vi "Konfig AK.vi"() -> ()   [LabVIEW 2020, in "AK-Schnittstelle.lvlib"]
uses:
  AK-Schnittstelle.lvlib
  Visualisierungs Elemente/VISA Control.ctl
  Seriell - Parity Bits.ctl
  Seriell - Stop Bits.ctl
  Seriell - Flow Control.ctl
  Visualisierungs Elemente/Button.ctl
  Seriell - Baud Rate.ctl
  Seriell - Data Bits.ctl
  Visualisierungs Elemente/String - Ausgabefeld.ctl
  AK Befehlssatz.ctl
  Aktionen Gespeicherte Werte.ctl
  Seiten/FT-IR/FGV FT-IR Gasliste Aktionen.ctl
  AK Namen Aktionen.ctl
  Daten weitergeben Aktionen.ctl
  SysLog/SysLog Interface.ctl
  Seiten/FT-IR/FT-IR.lvlib
  Allgemein/allgemeine Sub-VIs.lvlib
  Sprachverwaltung/Sprachverwaltung.lvlib
  SysLog/SysLog.lvlib
  <vilib>/Utility/Data Type/NI_Data Type.lvlib
  AK Seriell/AK Seriell.lvlib
panel:
  in  "Registerkarte":T1(tab)
  in  "Nur im Messen übertragen":bool caption="Loggen?"
  in  "AK Befehlssatz":T2=enum."AVL (Puma)"
  in  "Timeout":u16
  in  "Loggen?":bool
  in  "data bits":T3=8 items=["8"=8, "7"=7, "6"=6, "5"=5, "4"=4]
  in  "Baud Rate":T4=38400 items=["38400"=38400, "19200"=19200, "14400"=14400, "9600"=9600, "4800"=4800, "2400"=2400]
  in  "TCP aktiv":bool
  in  "Seriell aktiv":bool
  in  "Port":u16
  in  "flow control":T5 items=["None"=0, "XON/XOFF"=1, "RTS/CTS"=2, "DTR/DSR"=4]
  in  "stop bits":T6=10 items=["1.0"=10, "1.5"=15, "2.0"=20]
  in  "parity":T7 items=["None", "Odd", "Even", "Mark", "Space"]
  in  "VISA resource name":T8="COM1"
  out "EKFG vom Host":string[](array[string])
  in  "Original Liste":i32(listbox)
  in  "Konfigurierte Liste":i32(listbox)
  in  "Übernehmen":T9
  in  "Löschen":T9
  in  "Alle Löschen":T9
  in  "AK Namen":T10[](array[typedef])
  out "Gasliste":T10[](array[typedef])
  in  "Neuer Eintrag":T9
  out "Empfangspuffer":string[](array[string])
  out "Antwort":string[](array[string])
  out "Details ALLE":string[](array[string])
  in  "ABBRECHEN":T9
  in  "Speichern":T9
  # "Konfiguration AK-Schnittstelle"
  # "Seriell"
  # "TCP"
  # "Serielle Schnittstelle:"
  # "Port:"
  # "Baud rate:"
  # "Timeout:"
  # "sec"
  # "Data bits:"
  # "Parity bits:"
  # "Stop bits:"
  # "Flow control:"
  # "Messwerte nur in Messen übertragen:"
  # "AK in Datei Loggen:"
  # "AK Befehlssatz:"
  # "Konfiguration Kanalreihenfolge (EKFG)"
  # "Konfiguration AK-Namen (für EKFG)"
  # "Gasliste"
  # "AK Namen"
  # "Status AK-Kommunikation"
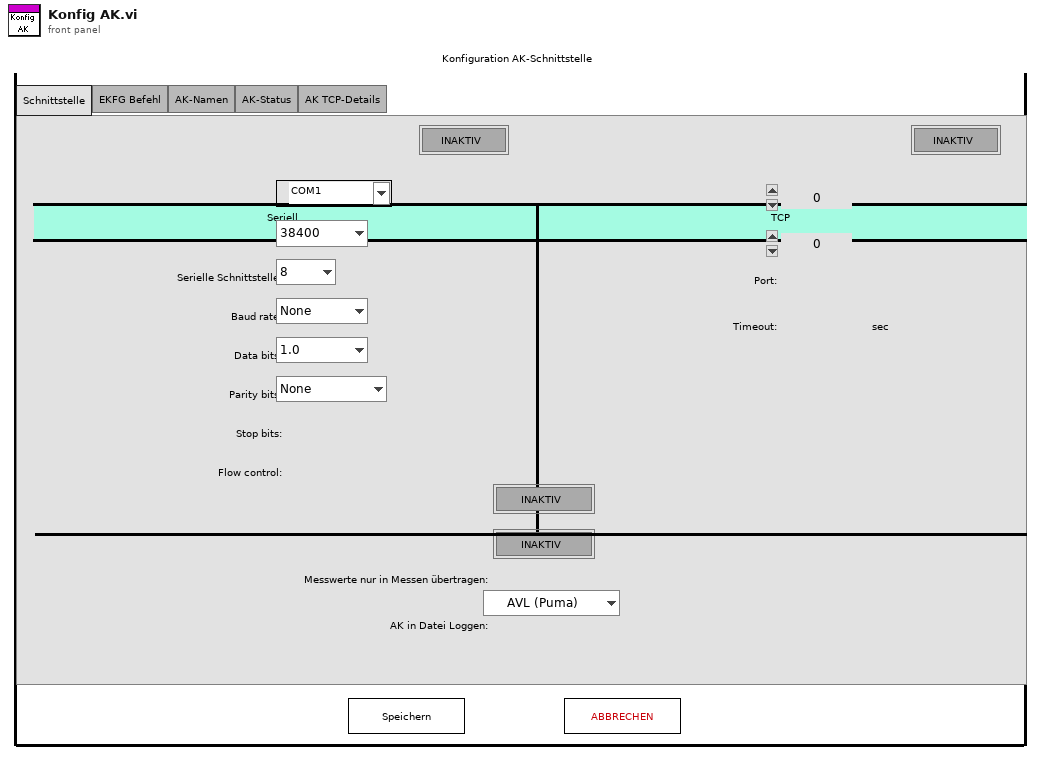
[diagram p1: front panel]
types:
  T1 = enum32{"Interface", "EKFG Commando", "AK-Name", "AK-Status", "AK TCP-Details"}
  T2 = typedef "AK-Schnittstelle.lvlib/AK Befehlssatz.ctl" = enum16{"MEXA", "IAG v1.4", "AVL (Puma)", "PEUS"}
  T3 = typedef "AK-Schnittstelle.lvlib/AK Seriell.lvlib/Seriell - Data Bits.ctl" = u16
  T4 = typedef "AK-Schnittstelle.lvlib/AK Seriell.lvlib/Seriell - Baud Rate.ctl" = u16
  T5 = typedef "AK-Schnittstelle.lvlib/AK Seriell.lvlib/Seriell - Flow Control.ctl" = u16
  T6 = typedef "AK-Schnittstelle.lvlib/AK Seriell.lvlib/Seriell - Stop Bits.ctl" = u16
  T7 = typedef "AK-Schnittstelle.lvlib/AK Seriell.lvlib/Seriell - Parity Bits.ctl" = u16
  T8 = typedef "VISA Control.ctl" = refnum<visa-resource-name>
  T9 = typedef "Button.ctl" = bool
  T10 = typedef "String - Ausgabefeld.ctl" = string
  T11 = typedef "FT-IR.lvlib/FGV FT-IR Gasliste Aktionen.ctl" = enum16{"lesen", "Gasliste FT-IR", "Gasliste ausgelesen", "laden", "speichern", "löschen"}
  T12 = typedef "AK-Schnittstelle.lvlib/AK Namen Aktionen.ctl" = enum16{"lesen", "laden", "speichern Namen", "AK Namen", "Liste erstellen", "EKFG erstellen", "speichern EKFG", "EKFG schreiben", "Neuen Eintrag erzeugen"}
  T13 = typedef "AK-Schnittstelle.lvlib/Aktionen Gespeicherte Werte.ctl" = enum16{"lesen", "laden", "speichern", "Seriell", "TCP", "Diverse", "AKTIV", "AK-Namen"}
  T14 = typedef "AK-Schnittstelle.lvlib/Diverse gespeicherte Werte.ctl" = cluster{"Kalibriergaseingang":i16, "SamplePoint":i16, "CalGas zu PNS":i16, "Gas-Reihenfolge":i16[], "Zeit 0-Gas":sgl, "Zeit CalGas":sgl, "AK Befehlssatz":T2}
  T15 = typedef "AK-Schnittstelle.lvlib/AK TCP.lvlib/TCP Parameter.ctl" = cluster{"Port":u16, "Timeout":u16}
  T16 = typedef "AK-Schnittstelle.lvlib/AK Seriell.lvlib/Serielle Parameter.ctl" = cluster{"VISA resource name":refnum<visa-resource-name>, "baud rate":u32, "data bits":u16, "parity":u16, "stop bits":u16, "flow control":u16}
  T17 = typedef "AK-Schnittstelle.lvlib/Daten weitergeben Aktionen.ctl" = enum16{"lesen", "schreiben", "Log löschen", "Detail", "Detail löschen", "Speicher Freigeben"}
  T18 = typedef "SysLog.lvlib/SysLog Interface.ctl" = cluster{"FehlermeldungsCode":i32, "ErfolgsmeldungsCode":i32, "ParameterListenString":string, "Anzeige":bool, "SysLogIcon":enum16{"OK", "Warnung", "Fehler"}, "intern":bool}
  T19 = typedef "AK-Schnittstelle.lvlib/AK Namen Listen.ctl" = cluster{"Namen":string[], "AK Namen":string[]}
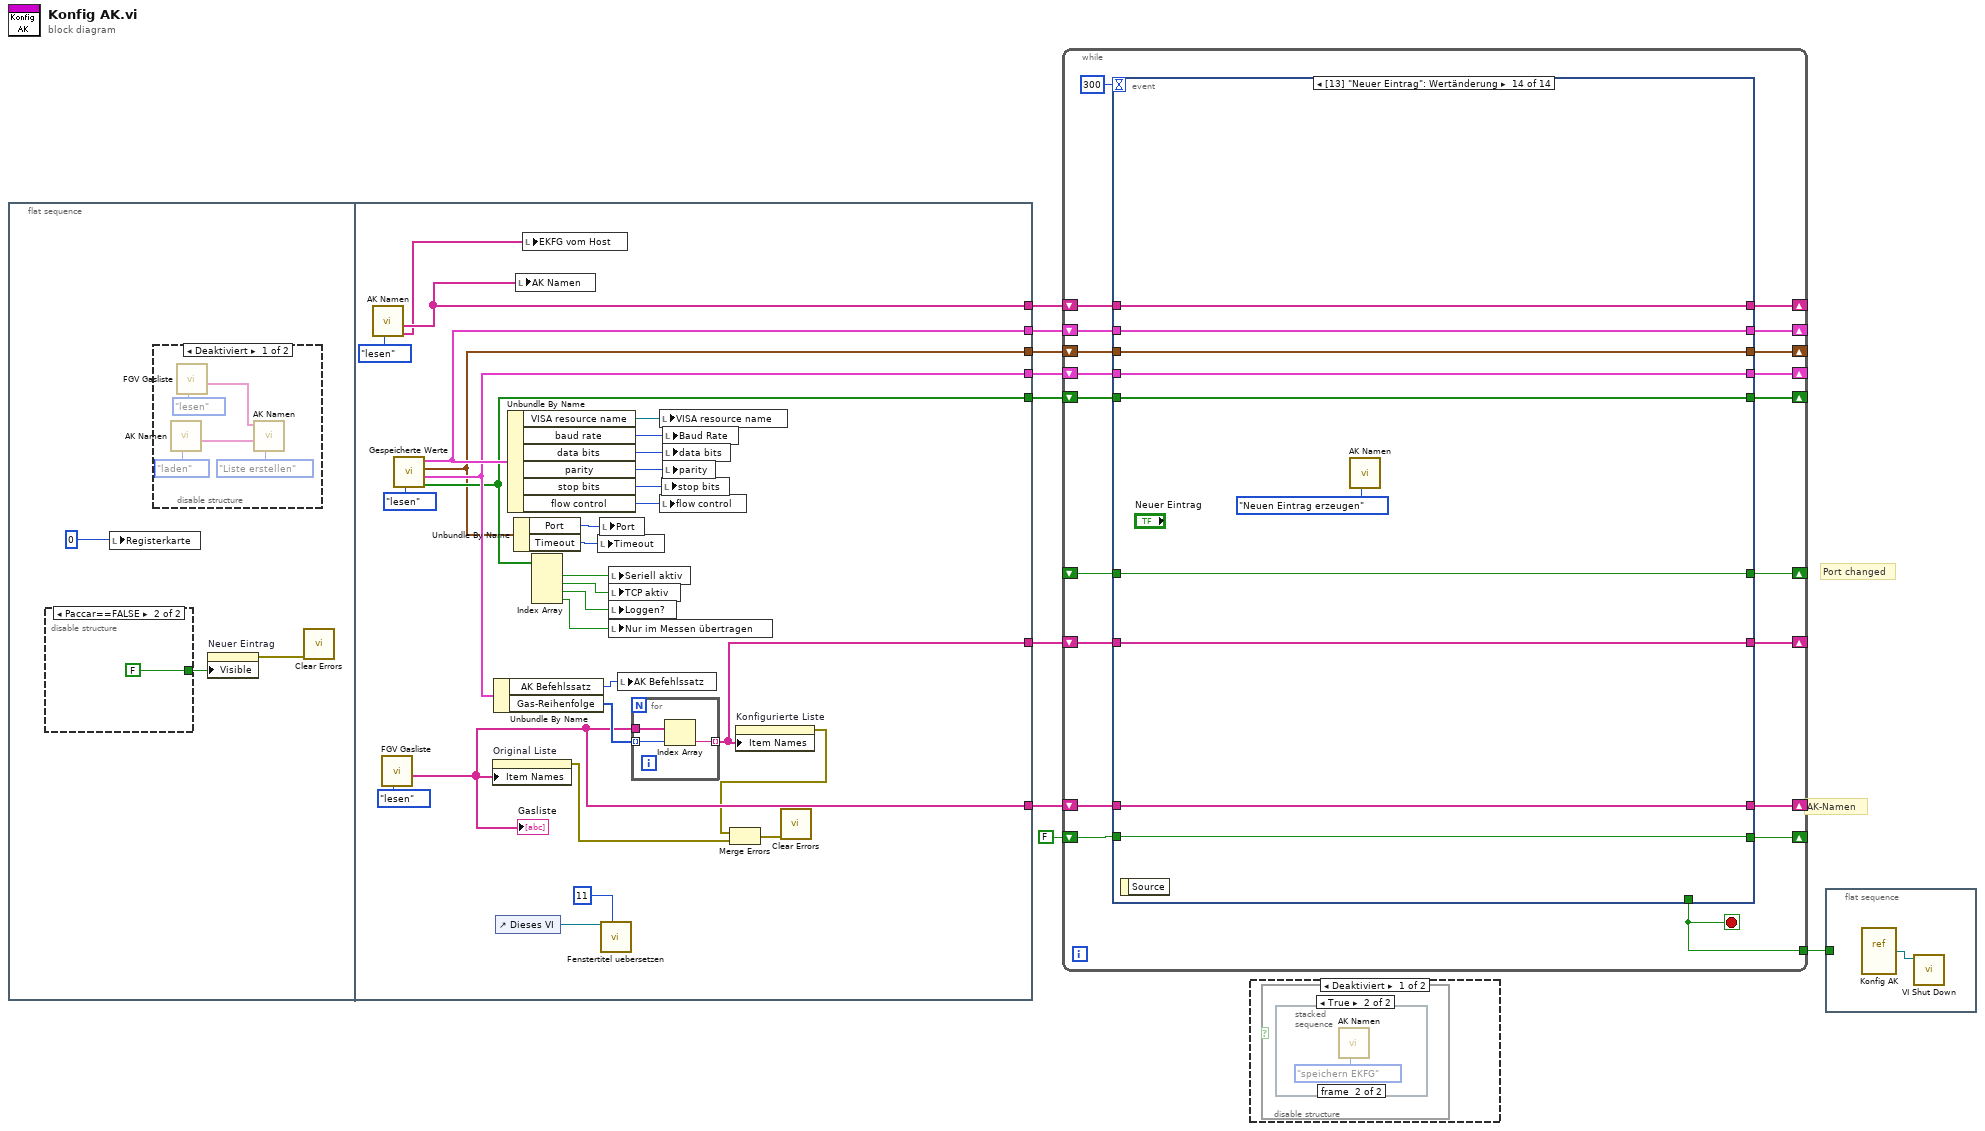
[diagram p0: block diagram]
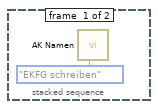
[diagram p3: hidden frame]
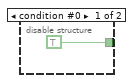
[diagram p5: hidden frame]
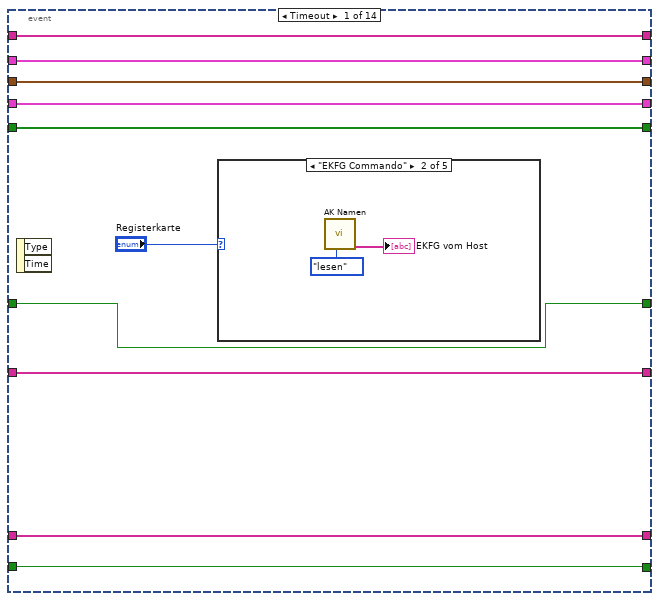
[diagram p7: hidden frame]
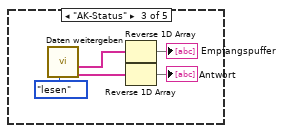
[diagram p9: hidden frame]
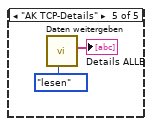
[diagram p11: hidden frame]
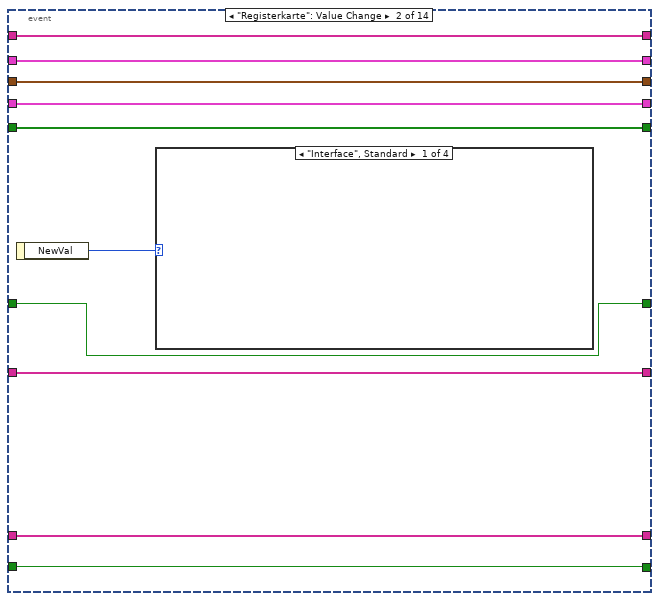
[diagram p12: hidden frame]
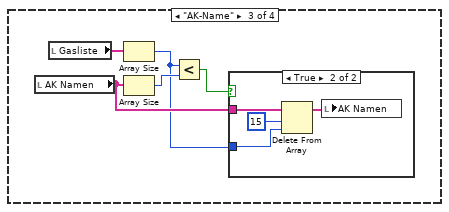
[diagram p14: hidden frame]
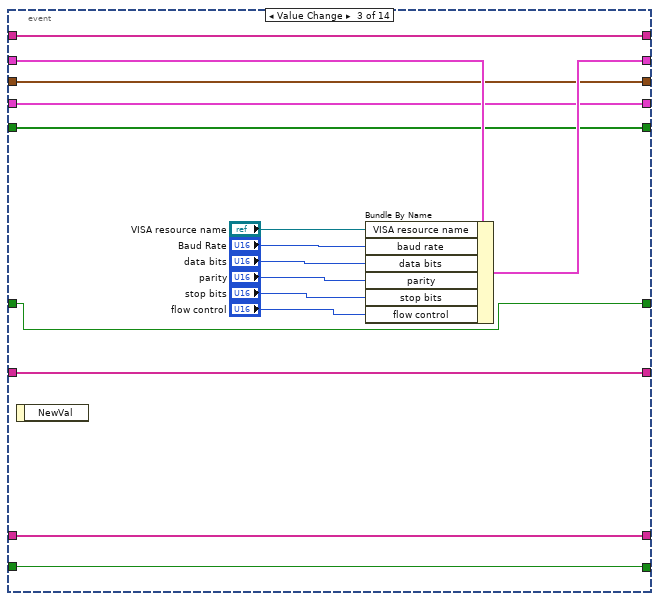
[diagram p17: hidden frame]
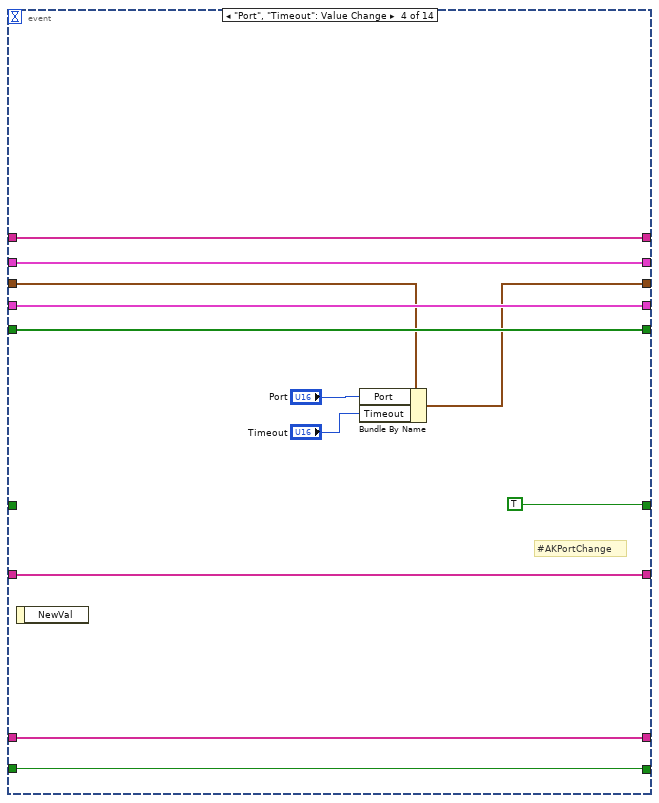
[diagram p18: hidden frame]
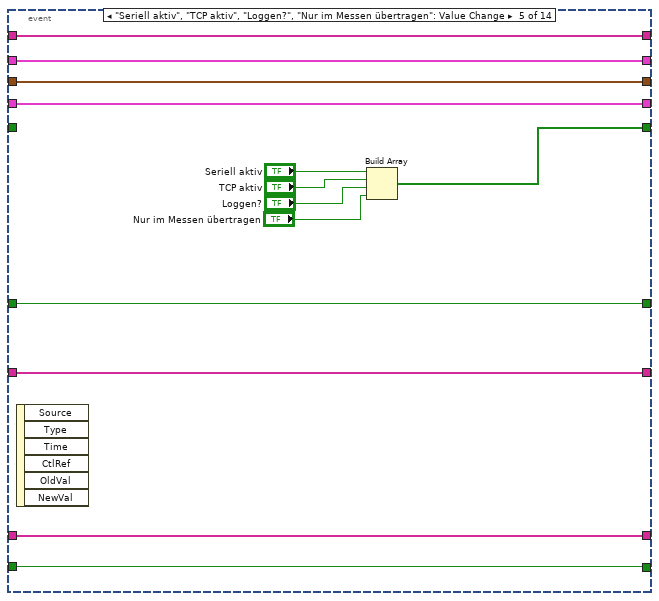
[diagram p19: hidden frame]
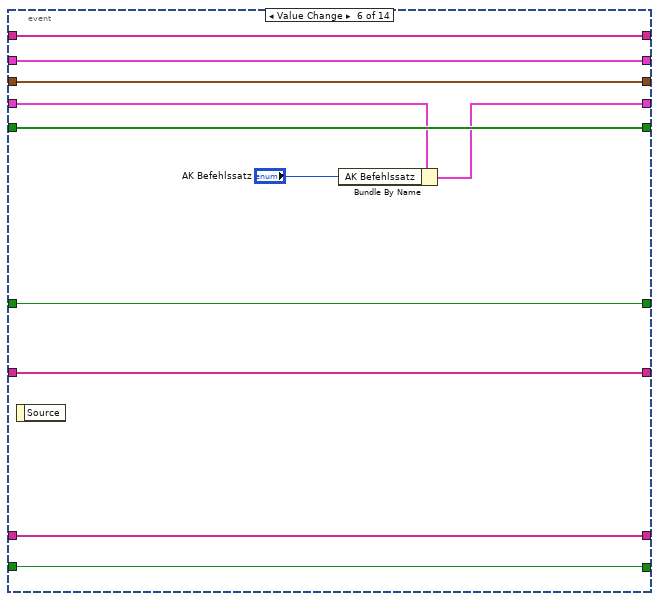
[diagram p20: hidden frame]
diagram:
  # "Port changed"
  # "AK-Namen"
  n1 = flat-sequence {
    tunnel: [w42] -> w9
    tunnel: [w33] -> w8
    tunnel: [w40] -> w7
    tunnel: [w38] -> w6
    tunnel: [w30] -> w4
    tunnel: [w35] -> w5
    tunnel: [w21] -> w3
    frame #0 {
      n2 = disable-structure shown="Paccar==FALSE" {
        disable-tunnel: [TRUE ("Sichtbar") FALSE ("Sichtbar")] -> w12
        frame condition #0 {
        }
        frame condition #1 (active) {
        }
      }
      n3 = local write "Registerkarte"(0) -> ()
      n4 = disable-structure shown="Deaktiviert" {
        frame Disabled {
          n5 = call "AK Namen.vi"("Aktionen"=AK_Namen_Aktionen."laden") -> ("AK Namen"=w17:string[])  [unwired: 7 in, 3 out]
          n6 = call "FGV Gasliste.vi"("Aktionen"=FGV_FT-IR_Gasliste_Aktionen."lesen") -> ("Aktuelle Gasliste gesamt"=w15:T10[])  [unwired: 8 in, 2 out]
          n7 = call "AK Namen.vi"("Aktionen"=AK_Namen_Aktionen."Liste erstellen", "AK Namen"=w17, "Aktuelle Gasliste FT-IR"=w15) -> ()  [unwired: 5 in, 4 out]
        }
        frame Enabled {
        }
      }
      n8 = property on="Neuer Eintrag" class="Bool."("Visible"=w12) -> (error out=w11:errorcluster)  [unwired: 2 in, 1 out]
      n9 = call <vilib>:"Clear Errors.vi"("error in (no error)"=w11) -> ()  [unwired: 5 in, 2 out]
    }
    frame #1 {
      n10 = call "AK Namen.vi"("Aktionen"=AK_Namen_Aktionen."lesen") -> ("EKFG Liste"=w20:string[], "AK Namen"=w21:string[])  [unwired: 7 in, 2 out]
      n11 = call "FGV Gasliste.vi"("Aktionen"=FGV_FT-IR_Gasliste_Aktionen."lesen") -> ("Aktuelle Gasliste gesamt"=w30:T10[])  [unwired: 8 in, 2 out]
      "Gasliste" <- w30
      n12 = call "Gespeicherte Werte.vi"("Aktionen"=Aktionen_Gespeicherte_Werte."lesen") -> ("AKTIV?"=w35:bool[], "Diverse Werte"=w40:T14, "TCP Parameter"=w33:T15, "Serielle Parameter"=w42:T16)  [unwired: 6 in, 1 out]
      n13 = property on="Original Liste" class="Listenfeld (strikt)"("Item Names"=w30) -> (error out=w27:errorcluster)  [unwired: 2 in, 1 out]
      n14 = Unbundle By Name(w40) -> ("AK Befehlssatz"=w29:T2, "Gas-Reihenfolge"=w39:i16[])
      n15 = control-ref of="Dieses VI"() -> (w24:refnum<vi>)
      n16 = Unbundle By Name(w42) -> ("VISA resource name"=w48:refnum<visa-resource-name>, "baud rate"=w47:u32, "data bits"=w46:u16, "parity"=w45:u16, "stop bits"=w44:u16, "flow control"=w43:u16)
      n17 = Unbundle By Name(w33) -> ("Port"=w32:u16, "Timeout"=w31:u16)
      n18 = local write "AK Namen"(w21) -> ()
      n19 = local write "EKFG vom Host"(w20) -> ()
      n20 = Index Array(array=w35) -> (element #1=w37:bool, element #2=w36:bool, element #3=w34:bool, element #4=w25:bool)  [unwired: 4 in]
      n21 = local write "Timeout"(w31) -> ()
      n22 = local write "Port"(w32) -> ()
      n23 = call "Fenstertitel uebersetzen.vi"("Index (Seite)"=11, "Dieses VI"=w24) -> ()  [unwired: 6 in, 4 out]
      n24 = local write "Seriell aktiv"(w37) -> ()
      n25 = local write "TCP aktiv"(w36) -> ()
      n26 = local write "Loggen?"(w34) -> ()
      n27 = local write "Nur im Messen übertragen"(w25) -> ()
      n28 = local write "AK Befehlssatz"(w29) -> ()
      n29 = for {
        tunnel: w39 -> [w52] mode=indexing
        tunnel: w30 -> [w51]
        tunnel: [w50] -> w38 mode=indexing
        n30 = Index Array(array=w51, index=w52) -> (element=w50:T10)
      }
      n31 = local write "VISA resource name"(w48) -> ()
      n32 = local write "flow control"(w43) -> ()
      n33 = local write "stop bits"(w44) -> ()
      n34 = local write "Baud Rate"(w47) -> ()
      n35 = local write "data bits"(w46) -> ()
      n36 = local write "parity"(w45) -> ()
      n37 = property on="Konfigurierte Liste" class="Listenfeld (strikt)"("Item Names"=w38) -> (error out=w28:errorcluster)  [unwired: 2 in, 1 out]
      n38 = Merge Errors(w28, w27) -> (w26:errorcluster)
      n39 = call <vilib>:"Clear Errors.vi"("error in (no error)"=w26) -> ()  [unwired: 5 in, 2 out]
    }
  }
  n40 = while {
    shift-right: [w70] -> _
    shift-left: w9 -> [w71]
    shift-right: [w67] -> _
    shift-left: w8 -> [w69]
    shift-right: [w66] -> _
    shift-left: w7 -> [w68]
    shift-right: [w64] -> _
    shift-left: w6 -> [w65]
    shift-right: [w62] -> _
    shift-left: w5 -> [w63]
    shift-right: [w61] -> _
    shift-left: w4 -> [w60]
    shift-right: [w58] -> _
    shift-left: w3 -> [w59]
    tunnel: [w57] -> w2
    shift-right: [w56] -> _
    shift-left: FALSE -> [w55]
    shift-right: [w54] -> _
    shift-left: _ -> [w53]
    stop <- w57 stop-if-true
    n41 = event shown="[13] \"Neuer Eintrag\": Wertänderung" {
      selector: _ -> [_ _ _ _ _ _ _ _ _ _ _ _ _ _]
      dyn-events: _ -> [_ _ _ _ _ _ _ _ _ _ _ _ _ _]
      timeout: 300 -> [_ _ _ _ _ _ _ _ _ _ _ _ _ _]
      tunnel: w71 -> [w82 w97 w126 w138 w148 w161 w176 w207 w221 w236 w253 w283 w309 w312]
      tunnel: [w82 w97 w125 w138 w148 w161 w176 w207 w221 w236 w253 w283 w309 w312] -> w70
      tunnel: [_ _ _ _ _ _ _ _ _ _ _ TRUE ("ABBRECHEN") TRUE ("ABBRECHEN") _] -> w57
      tunnel: w69 -> [w81 w96 w119 w133 w147 w160 w175 w206 w220 w235 w252 w282 w307 w313]
      tunnel: w68 -> [w80 w95 w120 w137 w146 w156 w172 w203 w217 w233 w251 w259 w306 w314]
      tunnel: [w81 w96 w119 w130 w147 w160 w175 w206 w220 w235 w252 w282 w307 w313] -> w67
      tunnel: [w80 w95 w120 w137 w146 w154 w171 w202 w216 w232 w251 w259 w306 w314] -> w66
      tunnel: w65 -> [w74 w100 w118 w136 w149 w158 w170 _ w219 _ w249 w277 w305 w316]
      tunnel: [w74 w100 w118 w136 w149 w158 w173 w205 w215 w231 w249 w277 w305 w316] -> w64
      tunnel: w63 -> [w79 w94 w117 w135 _ w159 w167 w201 w213 w230 w250 w274 w304 w315]
      tunnel: [w79 w94 w117 w135 w145 w159 w167 w201 w213 w230 w250 w274 w304 w315] -> w62
      tunnel: [w77 w99 w114 w134 w144 w157 w166 w200 w212 w229 w248 w273 w303 w317] -> w61
      tunnel: w60 -> [w77 w99 w114 w134 w144 w157 w166 w200 w212 w229 w248 w273 w303 w317]
      tunnel: w59 -> [w76 w98 w113 w129 w142 w162 w165 w199 w211 w228 _ w271 w302 w311]
      tunnel: [w76 w98 w113 w129 w142 w162 w165 w199 w211 w228 w242 w271 w302 w311] -> w58
      tunnel: [w75 w93 w112 w128 w140 w153 TRUE TRUE TRUE TRUE w241 w266 w301 w319] -> w56
      tunnel: w55 -> [w75 w93 w112 w128 w140 w153 _ _ _ _ w241 w266 w301 w319]
      tunnel: [w73 w92 w111 TRUE w139 w152 w163 w196 w208 w225 w240 FALSE w300 w318] -> w54
      tunnel: w53 -> [w73 w92 w111 _ w139 w152 w163 w196 w208 w225 w240 w260 w300 w318]
      event Timeout {
        n42 = event-data() -> ()  [unwired: 1 in, 2 out]
        n43 = case shown="\"EKFG Commando\"" "Registerkarte" {
          frame "Interface", Default {
          }
          frame "EKFG Commando" {
            n44 = call "AK Namen.vi"("Aktionen"=AK_Namen_Aktionen."lesen") -> ("EKFG Liste"=→"EKFG vom Host":string[])  [unwired: 7 in, 3 out]
          }
          frame "AK-Status" {
            n45 = call "Daten weitergeben.vi"("Aktionen"=Daten_weitergeben_Aktionen."lesen") -> ("Antwort"=w86:string[], "Empfangspuffer"=w88:string[])  [unwired: 6 in, 3 out]
            n46 = Reverse 1D Array(array=w88) -> (reversed array=→"Empfangspuffer":string[])
            n47 = Reverse 1D Array(array=w86) -> (reversed array=→"Antwort":string[])
          }
          frame "AK-Name" {
          }
          frame "AK TCP-Details" {
            n48 = call "Daten weitergeben.vi"("Aktionen"=Daten_weitergeben_Aktionen."lesen") -> ("Details ALLE"=→"Details ALLE":string[])  [unwired: 6 in, 4 out]
          }
        }
      }
      event "Registerkarte": Value Change {
        n49 = event-data() -> ("NewVal"=w101:T1)  [unwired: 1 in]
        n50 = case shown="\"Interface\", Standard" w101 {
          frame "Interface", Default {
          }
          frame "EKFG Commando" {
          }
          frame "AK-Name" {
            n51 = local read "AK Namen"() -> (w104:T10[])
            n52 = local read "Gasliste"() -> (w106:T10[])
            n53 = Array Size(array=w106) -> (size(s)=w103:i32)
            n54 = Array Size(array=w104) -> (size(s)=w105:i32)
            n55 = Less?(x=w103, y=w105) -> (x < y?=w102:bool)
            n56 = case shown="True" w102 {
              tunnel: w104 -> [_ w110]
              tunnel: w103 -> [_ w107]
              frame False {
              }
              frame True {
                n57 = Delete From Array(array=w110, length=15 ("Länge"), index=w107) -> (array with subset deleted=w108:T10[])  [unwired: 1 out]
                n58 = local write "AK Namen"(w108) -> ()
              }
            }
          }
          frame "AK-Status" {
          }
        }
      }
      event Value Change {
        n59 = event-data() -> ()  [unwired: 1 in, 1 out]
        n60 = Bundle By Name(cluster=w126, "VISA resource name"="VISA resource name", "baud rate"="Baud Rate", "data bits"="data bits", "parity"="parity", "stop bits"="stop bits", "flow control"="flow control") -> (w125:T16)
      }
      event "Port", "Timeout": Value Change {
        # "#AKPortChange"
        n61 = event-data() -> ()  [unwired: 1 in, 1 out]
        n62 = Bundle By Name(cluster=w133, "Port"="Port", "Timeout"="Timeout") -> (w130:T15)
      }
      event "Seriell aktiv", "TCP aktiv", "Loggen?", "Nur im Messen übertragen": Value Change {
        n63 = event-data() -> ()  [unwired: 1 in, 6 out]
        n64 = Build Array("Seriell aktiv", "TCP aktiv", "Loggen?", "Nur im Messen übertragen") -> (w145:bool[])
      }
      event Value Change {
        n65 = event-data() -> ()  [unwired: 1 in, 1 out]
        n66 = Bundle By Name(cluster=w156, "AK Befehlssatz"="AK Befehlssatz") -> (w154:T14)
      }
      event Value Change {
        n67 = event-data() -> ()  [unwired: 1 in, 1 out]
        n68 = Index Array(array=w166, index="Original Liste") -> (element=w169:T10)
        n69 = for {
          tunnel: w170 -> [w182] mode=indexing
          tunnel: w169 -> [w181]
          tunnel: [w177] -> w168
          stop <- w177 stop-if-true
          n70 = Not Equal?(x="AK DUMMY", y=w181) -> (x != y?=w179:bool)
          n71 = Equal?(x=w182, y=w181) -> (x = y?=w178:bool)
          n72 = And(x=w179, y=w178) -> (x .and. y?=w177:bool)
        }
        n73 = case shown="False" w168 {
          tunnel: w170 -> [w190 w194]
          tunnel: w169 -> [w189 _]
          tunnel: w166 -> [w188 _]
          tunnel: [w187 w194] -> w173
          tunnel: w172 -> [w186 w195]
          tunnel: [w185 w195] -> w171
          frame False {
            n74 = Build Array (concatenate)(w190, w189) -> (w187:T10[])
            n75 = for {
              tunnel: w188 -> [w193]
              tunnel: w187 -> [w192] mode=indexing
              tunnel: [w191] -> w184 mode=indexing
              n76 = Search 1D Array(1D array=w193, element=w192) -> (index of element=w191:i32)  [unwired: 1 in]
            }
            n77 = property on="Konfigurierte Liste" class="Listenfeld (strikt)"("Item Names"=w187) -> (error out=w183:errorcluster)  [unwired: 2 in, 1 out]
            n78 = Bundle By Name(cluster=w186, "Gas-Reihenfolge"=w184) -> (w185:T14)
            n79 = call <vilib>:"Clear Errors.vi"("error in (no error)"=w183) -> ()  [unwired: 5 in, 2 out]
          }
          frame True {
          }
        }
      }
      event Value Change {
        w205 = string[] [] ("Objektnamen")
        n80 = event-data() -> ()  [unwired: 1 in, 1 out]
        n81 = Bundle By Name(cluster=w203, "Gas-Reihenfolge"=i16[] []) -> (w202:T14)
        n82 = property on="Konfigurierte Liste" class="Listenfeld (strikt)"("Item Names"=w205) -> (error out=w198:errorcluster)  [unwired: 2 in, 1 out]
        n83 = call <vilib>:"Clear Errors.vi"("error in (no error)"=w198) -> ()  [unwired: 5 in, 2 out]
      }
      event Value Change {
        n84 = event-data() -> ()  [unwired: 1 in, 1 out]
        n85 = local read "Konfigurierte Liste"() -> (w214:i32)
        n86 = Delete From Array(array=w219, index=w214) -> (array with subset deleted=w215:T10[])  [unwired: 1 in, 1 out]
        n87 = for {
          tunnel: w212 -> [w224]
          tunnel: w215 -> [w223] mode=indexing
          tunnel: [w222] -> w218 mode=indexing
          n88 = Search 1D Array(1D array=w224, element=w223) -> (index of element=w222:i32)  [unwired: 1 in]
        }
        n89 = Bundle By Name(cluster=w217, "Gas-Reihenfolge"=w218) -> (w216:T14)
        n90 = property on="Konfigurierte Liste" class="Listenfeld (strikt)"("Item Names"=w215) -> (error out=w210:errorcluster)  [unwired: 2 in, 1 out]
        n91 = call <vilib>:"Clear Errors.vi"("error in (no error)"=w210) -> ()  [unwired: 5 in, 2 out]
      }
      event "Konfigurierte Liste": Drag Ended {
        n92 = event-data() -> ()  [unwired: 1 in, 1 out]
        n93 = property on="Konfigurierte Liste" class="Listenfeld (strikt)"() -> (error out=w227:errorcluster, "Item Names"=w231:string[])  [unwired: 2 in, 1 out]
        n94 = call <vilib>:"Clear Errors.vi"("error in (no error)"=w227) -> ()  [unwired: 5 in, 2 out]
        n95 = for {
          tunnel: w229 -> [w239]
          tunnel: w231 -> [w238] mode=indexing
          tunnel: [w237] -> w234 mode=indexing
          n96 = Search 1D Array(1D array=w239, element=w238) -> (index of element=w237:i32)  [unwired: 1 in]
        }
        n97 = Bundle By Name(cluster=w233, "Gas-Reihenfolge"=w234) -> (w232:T14)
      }
      event "AK Namen": Value Change {
        n98 = event-data() -> ()  [unwired: 1 in, 1 out]
        n99 = local read "Gasliste"() -> (w247:T10[])
        n100 = Array Size(array=w247) -> (size(s)=w245:i32)
        n101 = Array Size(array="AK Namen") -> (size(s)=w246:i32)
        n102 = Less?(x=w245, y=w246) -> (x < y?=w244:bool)
        n103 = case shown="True" w244 {
          tunnel: "AK Namen" -> [w254 w258]
          tunnel: w245 -> [_ w256]
          tunnel: [w254 w255] -> w242
          frame False {
          }
          frame True {
            n104 = Delete From Array(array=w258, length=15 ("Länge"), index=w256) -> (array with subset deleted=w255:T10[])  [unwired: 1 out]
            n105 = local write "AK Namen"(w255) -> ()
          }
        }
      }
      event Value Change {
        # "#AK_Fehler"
        # "AK-Namen"
        n106 = event-data() -> ()  [unwired: 1 in, 1 out]
        n107 = call "Gespeicherte Werte.vi"("Aktionen"=Aktionen_Gespeicherte_Werte."Seriell", "Serielle Parameter"=w283) -> ("Serielle Parameter"=w279:T16)  [unwired: 5 in, 4 out]
        n108 = Unbundle By Name(w259) -> ("AK Befehlssatz"=w262:T2)
        n109 = case shown="True" w266 {
          frame False {
          }
          frame True {
            n110 = stacked-sequence {
              frame #0 {
                n111 = call "AK Namen.vi"("Aktionen"=AK_Namen_Aktionen."EKFG schreiben") -> ()  [unwired: 7 in, 4 out]
              }
              frame #1 {
                n112 = call "AK Namen.vi"("Aktionen"=AK_Namen_Aktionen."speichern EKFG") -> ()  [unwired: 7 in, 4 out]
              }
            }
          }
        }
        n113 = call "Gespeicherte Werte.vi"("Port changed in"=w260, "Aktionen"=Aktionen_Gespeicherte_Werte."TCP", "TCP Parameter"=w282, "Serielle Parameter"=w279) -> ("Diverse Werte"=w264:T14, "Serielle Parameter"=w278:T16)  [unwired: 3 in, 3 out]
        n114 = Unbundle By Name(w264) -> ("AK Befehlssatz"=w265:T2)
        n115 = call "Gespeicherte Werte.vi"("Aktionen"=Aktionen_Gespeicherte_Werte."Diverse", "Diverse Werte"=w259, "Serielle Parameter"=w278) -> ("Serielle Parameter"=w275:T16)  [unwired: 4 in, 4 out]
        n116 = Not Equal?(x=w265, y=w262) -> (x != y?=w263:bool)
        n117 = case shown="True" w263 {
          tunnel: w262 -> [_ w287]
          frame False {
          }
          frame True {
            n118 = disable-structure shown="SysLogAktiv==TRUE" {
              disable-tunnel: w287 -> [w294 _]
              frame condition #0 (active) {
                n119 = call <vilib>:"Get Numeric Information.vi"("variant"=AK_Befehlssatz."IAG v1.4" ("AK Befehlssatz")) -> ("enum names"=w293:string[])  [unwired: 7 in, 3 out]
                n120 = Index Array(array=w293, index=w294) -> (element=w288:string)
                n121 = Bundle By Name(cluster=T18 {"FehlermeldungsCode"=9, "ErfolgsmeldungsCode"=9, "ParameterListenString"="", "Anzeige"=TRUE, "SysLogIcon"=enum."OK", "intern"=FALSE} ("Cluster (in)"), "ParameterListenString"=w288) -> (w289:T18)
                n122 = call "Syslog Interface PC.vi"("Fehler (in)"=errorcluster {"status"=FALSE, "code"=0, "source"=""}, "Cluster (in)"=w289) -> ()  [unwired: 9 in, 1 out]
              }
              frame condition #1 {
              }
            }
          }
        }
        n123 = call "Gespeicherte Werte.vi"("Aktionen"=Aktionen_Gespeicherte_Werte."AKTIV", "AKTIV?"=w274, "Serielle Parameter"=w275) -> ("Serielle Parameter"=w272:T16)  [unwired: 4 in, 4 out]
        n124 = flat-sequence {
          tunnel: w268 -> [_]
          frame #0 {
            n125 = call "FGV Gasliste.vi"("Aktionen"=FGV_FT-IR_Gasliste_Aktionen."lesen") -> ("Aktuelle Gasliste gesamt"=w297:T10[])  [unwired: 8 in, 2 out]
            n126 = call "AK Namen.vi"("Aktionen"=AK_Namen_Aktionen."Liste erstellen", "Aktuelle Gasliste FT-IR"=w297) -> ()  [unwired: 6 in, 4 out]
          }
        }
        n127 = call "AK Namen.vi"("Aktionen"=AK_Namen_Aktionen."AK Namen", "AK Namen"=w271) -> ("Namen"=w270:string[])  [unwired: 6 in, 3 out]
        n128 = call "Gespeicherte Werte.vi"("Aktionen"=Aktionen_Gespeicherte_Werte."speichern", "Serielle Parameter"=w272) -> ()  [unwired: 5 in, 5 out]
        n129 = call "AK Namen.vi"("Aktionen"=AK_Namen_Aktionen."speichern Namen", "Aktuelle Gasliste FT-IR"=w270) -> ("AK Namen Liste"=w268:T19)  [unwired: 6 in, 3 out]
      }
      event Value Change {
        n130 = event-data() -> ()  [unwired: 1 in, 1 out]
      }
      event Value Change {
        n131 = event-data() -> ()  [unwired: 1 in, 1 out]
        n132 = call "AK Namen.vi"("Aktionen"=AK_Namen_Aktionen."Neuen Eintrag erzeugen") -> ()  [unwired: 7 in, 4 out]
      }
    }
  }
  n133 = disable-structure shown="Deaktiviert" {
    frame Disabled {
      n134 = case shown="True" {
        selector: _ -> [_ _]
        frame False {
        }
        frame True {
          n135 = stacked-sequence {
            frame #0 {
              n136 = call "AK Namen.vi"("Aktionen"=AK_Namen_Aktionen."EKFG schreiben") -> ()  [unwired: 7 in, 4 out]
            }
            frame #1 {
              n137 = call "AK Namen.vi"("Aktionen"=AK_Namen_Aktionen."speichern EKFG") -> ()  [unwired: 7 in, 4 out]
            }
          }
        }
      }
    }
    frame Enabled {
    }
  }
  n138 = flat-sequence {
    tunnel: w2 -> [_]
    frame #0 {
      n139 = vi-ref "Konfig AK.vi"() -> (w322:refnum<vi>)
      n140 = call "VI Shut Down.vi"("VI Referenz"=w322) -> ()  [unwired: 11 in]
    }
  }
